vi "LCD Display Test.vi"(10 "Simulation Data":T1={"PowerOn"=TRUE, "Battery"=TRUE, "Antenna"=TRUE, "Microphone"=TRUE, "Speakers"=TRUE, "Buttons"=TRUE, "LCD"=enum."Passing Image"}, 11 "Test Image Name":string="LCD_Image_Test.png") -> (0 "error out":errorcluster, 1 "Image Report String":string, 2 "Number of Dead Pixels":dbl, 3 "Average Pixel Brightness Difference":dbl)   [LabVIEW 2011]
doc: "Measures the Test fixture microphone input while a frequency sweep test sound is played by the speaker on the UUT. The amplitude of the response is measured to ensure that the UUT speaker is playing all pitches in the desired frequency range. The Test returns the minimum measured amplitude of all tested frequencies."
uses:
  Support/Simulation Data.ctl
panel:
  out "Expected Test Image":picture
  out "Image Displayed on UUT":picture
  # "Settings"
  # "Results"
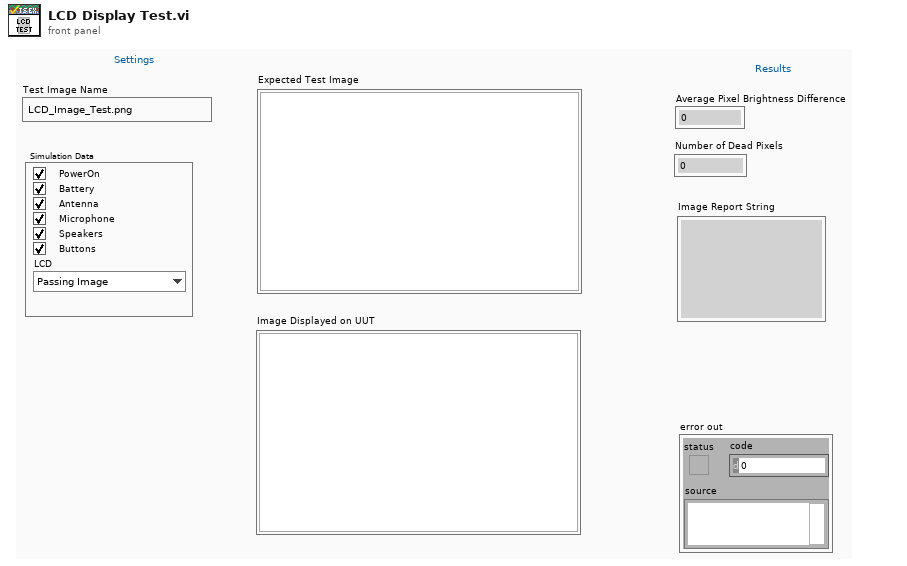
[diagram p1: front panel]
types:
  T1 = typedef "Simulation Data.ctl" = cluster{"PowerOn":bool, "Battery":bool, "Antenna":bool, "Microphone":bool, "Speakers":bool, "Buttons":bool, "LCD":enum16{"Passing Image", "Dead Pixels", "Incorrect Brightness"}}
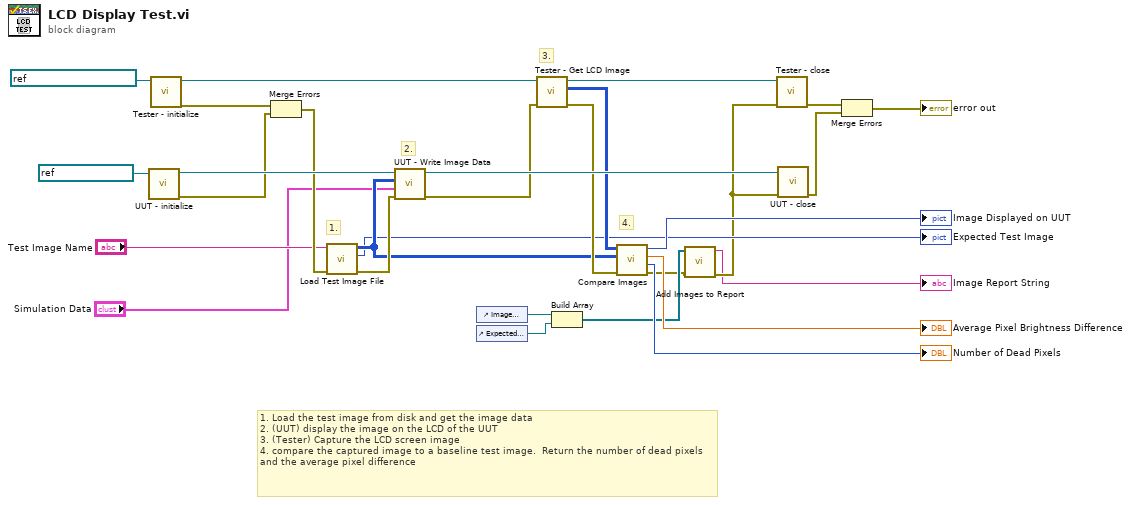
[diagram p0: block diagram]
diagram:
  # "1."
  # "4."
  # "3."
  # "2."
  # "1. Load the test image from disk and get the image data \n2. (UUT) display the image on the LCD of the UUT\n3. (Tester) Capture the LCD screen image\n4. compare the captured image to a baseline test image.  Return the number of dead pixels and the average pixel difference"
  n1 = call "UUT - initialize.vi"("VISA resource name"=refnum<visa-resource-name> "UUTController") -> ("error out"=w17:errorcluster, "VISA resource name out"=w27:refnum<visa-resource-name>)  [unwired: 9 in]
  n2 = call "Tester - initialize.vi"("VISA resource name"=refnum<visa-resource-name> "TesterVideoMeasure") -> ("error out"=w28:errorcluster, "VISA resource name out"=w26:refnum<visa-resource-name>)  [unwired: 9 in]
  n3 = Merge Errors(w28, w17) -> (w16:errorcluster)
  n4 = call "Load Test Image File.vi"("error in (no error)"=w16, "name or relative path"="Test Image Name") -> ("error out"=w15:errorcluster, "Test Image"=→"Expected Test Image":picture, "Test Image Data"=w14:u32[][])  [unwired: 7 in]
  n5 = call "UUT - Write Image Data.vi"("error in (no error)"=w15, "Simulation Data"="Simulation Data", "Test Image Data"=w14, "VISA resource name"=w27) -> ("error out"=w20:errorcluster, "VISA resource name out"=w23:refnum<visa-resource-name>)  [unwired: 6 in]
  n6 = control-ref of="Image Displayed on UUT"() -> (w6:refnum<vi>)
  n7 = control-ref of="Expected Test Image"() -> (w5:refnum<vi>)
  n8 = call "Tester - Get LCD Image.vi"("error in (no error)"=w20, "VISA resource name"=w26) -> ("error out"=w18:errorcluster, "24-bit pixmap"=w19:u32[][], "VISA resource name out"=w24:refnum<visa-resource-name>)  [unwired: 7 in]
  n9 = Build Array(w6, w5) -> (w4:refnum<vi>[])
  n10 = call "Compare Images.vi"("error in (no error)"=w18, "Test Image Data"=w14, "UUT Image Data"=w19) -> ("error out"=w3:errorcluster, "Number of Dead Pixels"=→"Number of Dead Pixels":i32, "Average Pixel Difference"=→"Average Pixel Brightness Difference":dbl, "UUT Image"=→"Image Displayed on UUT":picture)  [unwired: 5 in]
  n11 = call "Add Images to Report.vi"("error in (no error)"=w3, "Control References"=w4) -> ("error out"=w2:errorcluster, "Report String"=→"Image Report String":string)  [unwired: 8 in]
  n12 = call "Tester - close.vi"("error in (no error)"=w2, "VISA resource name"=w24) -> ("error out"=w21:errorcluster)  [unwired: 9 in]
  n13 = call "UUT - close.vi"("error in (no error)"=w2, "VISA resource name"=w23) -> ("error out"=w22:errorcluster)  [unwired: 9 in]
  n14 = Merge Errors(w21, w22) -> (→"error out":errorcluster)
